vi "Create lvclass Folder.vi"(9 "Name":string, 10 "Library Folder Path":path) -> (2 "Class Folder Path":path)   [LabVIEW 2021, in "_Create From Template.lvlib" / "Script Strategy.lvlib"]
uses:
  Script Strategy.lvlib
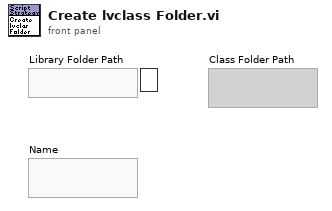
[diagram p1: front panel]
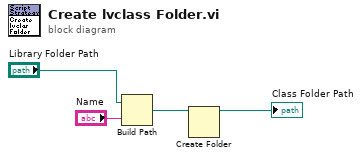
[diagram p0: block diagram]
diagram:
  n1 = Build Path(base path="Library Folder Path", name or relative path="Name") -> (appended path=w4:path)
  n2 = Create Folder(path (use dialog)=w4) -> (created path=→"Class Folder Path":path)  [unwired: 2 in, 2 out]
